vi "Sub_get_freq_bounds_FEA.vi"(2 "FEA Parameters":T1={"LEMP"={"Eigenvalues"=[], "Square Transpose Eigenvectors"=[], "1/deltaStiff"=0.0}, "nodes of interest"=[], "all nodes"=[], "Eigenvalue Method"=enum."0-Local Eigen Modification Procedure", "Mode Count"=3, "initial_pin_node"=0, "Sub Sample"=TRUE}, 3 "Modeling Parameters":T2) -> (0 "FEA Parameters":T1, 1 "Modeling Parameters":T2)   [LabVIEW 2021]
panel:
  out "Waveform Graph":dynamicdata(graph)
  out "third modes":dbl[](array[numeric])
  out "first modes":dbl[](array[numeric])
  out "second modes":dbl[](array[numeric])
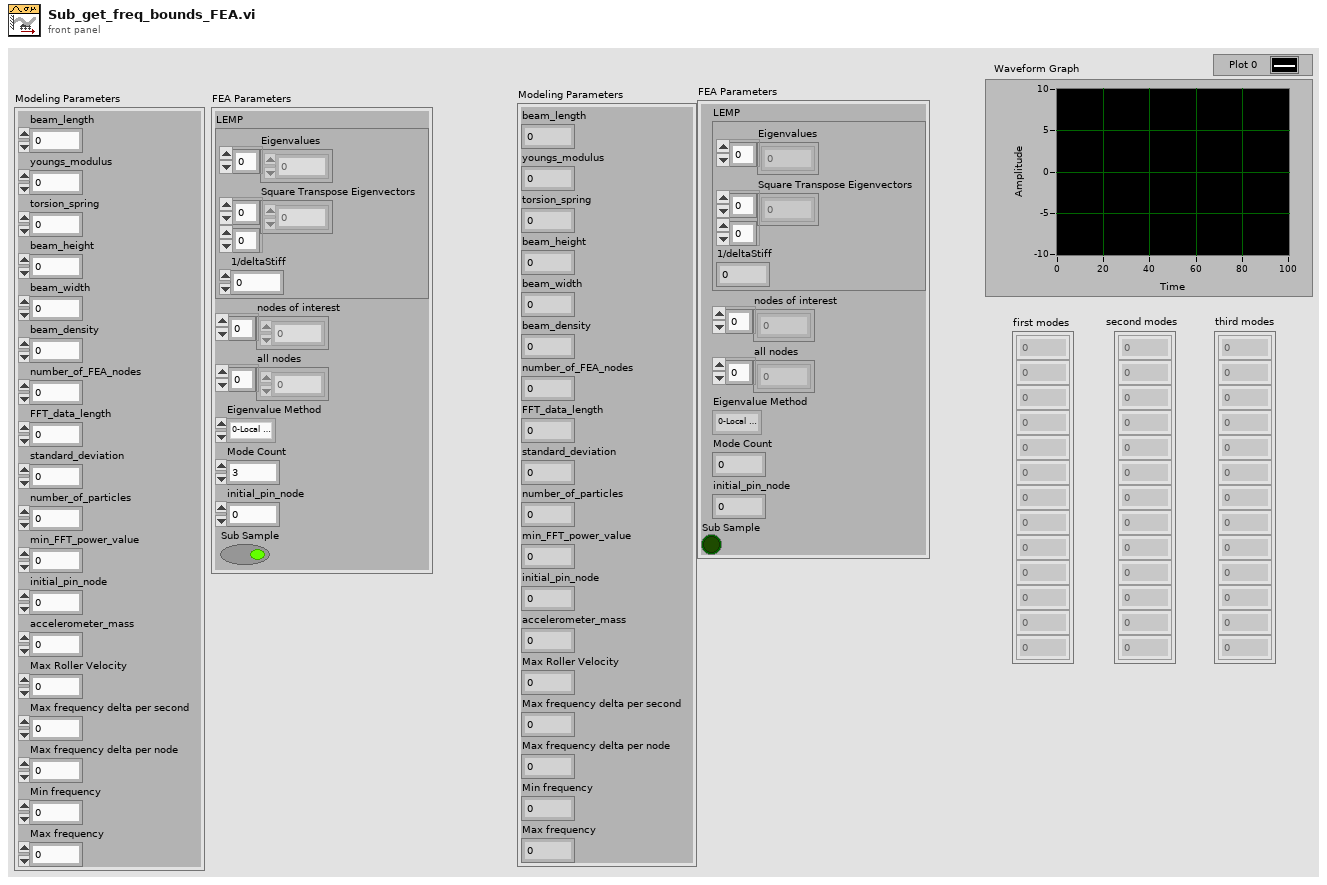
[diagram p1: front panel]
types:
  T1 = cluster{"LEMP":cluster{"Eigenvalues":dbl[], "Square Transpose Eigenvectors":dbl[][], "1/deltaStiff":dbl}, "nodes of interest":i32[], "all nodes":i32[], "Eigenvalue Method":enum16{"0-Local Eigen Modification Procedure", "1-LabVIEW generalized eigenvalues", "2-LabVIEW M^-1K eigenvalues", "3-LabVIEW Cholesky Factorization", "4-Cholesky Factorization CPU SGL", "5-Cholesky Factorization CPU FXP", "6-Cholesky Factorization FPGA SGL", "7-Cholesky Factorization FPGA SGL SCL"}, "Mode Count":i32, "initial_pin_node":i32, "Sub Sample":bool}
  T2 = cluster{"beam_length":dbl, "youngs_modulus":dbl, "torsion_spring":dbl, "beam_height":dbl, "beam_width":dbl, "beam_density":dbl, "number_of_FEA_nodes":i32, "FFT_data_length":i32, "standard_deviation":dbl, "number_of_particles":i32, "min_FFT_power_value":dbl, "initial_pin_node":i32, "accelerometer_mass":dbl, "Max Roller Velocity":dbl, "Max frequency delta per second":dbl, "Max frequency delta per node":dbl, "Min frequency":dbl, "Max frequency":dbl}
  T3 = cluster{"Eigenvalues":dbl[], "Square Transpose Eigenvectors":dbl[][], "1/deltaStiff":dbl}
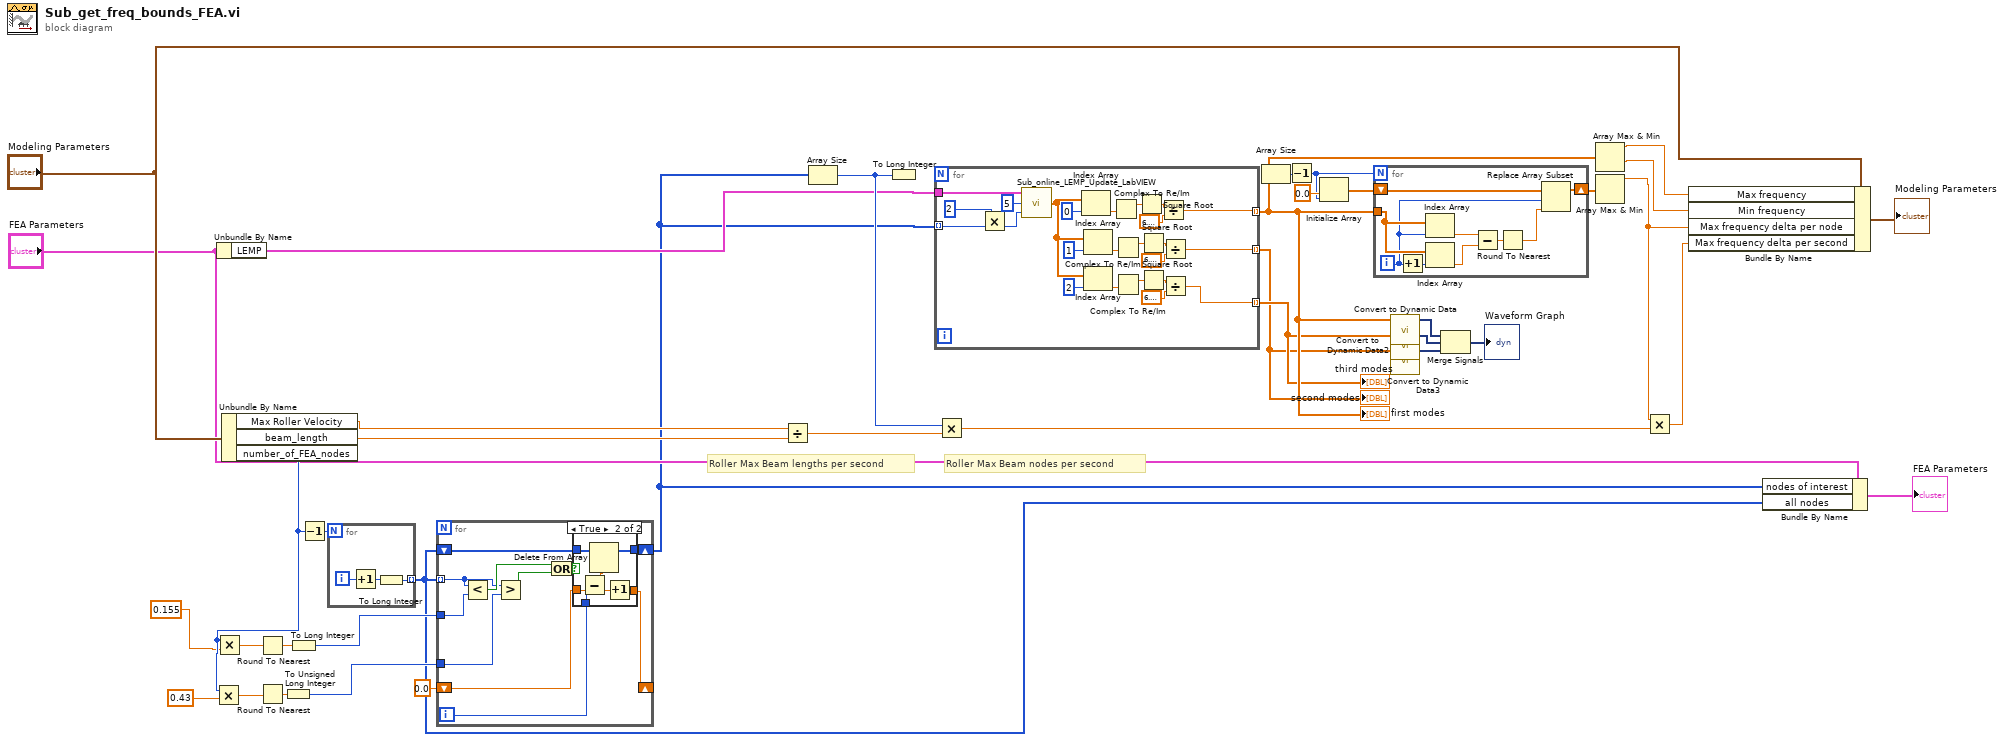
[diagram p0: block diagram]
diagram:
  # "Roller Max Beam nodes per second"
  # "Roller Max Beam lengths per second"
  n1 = Unbundle By Name("FEA Parameters") -> ("LEMP"=w12:T3)
  n2 = Unbundle By Name("Modeling Parameters") -> ("Max Roller Velocity"=w37:dbl, "beam_length"=w36:dbl, "number_of_FEA_nodes"=w29:i32)
  n3 = Multiply(x=w29, y=0.43) -> (x*y=w28:dbl)
  n4 = Multiply(x=w29, y=0.155) -> (x*y=w27:dbl)
  n5 = Round To Nearest(number=w27) -> (nearest integer value=w26:dbl)
  n6 = Round To Nearest(number=w28) -> (nearest integer value=w25:dbl)
  n7 = To Unsigned Long Integer(number=w25) -> (unsigned 32bit integer=w24:u32)
  n8 = To Long Integer(number=w26) -> (32bit integer=w23:i32)
  n9 = Decrement(x=w29) -> (x-1=w33:i32)
  n10 = for {
    N: w33 -> [_]
    tunnel: [w42] -> w19 mode=indexing
    i -> [w40]
    n11 = Increment(x=w40) -> (x+1=w41:i32)
    n12 = To Long Integer(number=w41) -> (32bit integer=w42:i32)
  }
  n13 = for {
    tunnel: w19 -> [w46] mode=indexing
    shift-right: [w49] -> w11
    shift-left: w19 -> [w53]
    shift-right: [w48] -> _
    shift-left: 0.0 -> [w47]
    tunnel: w23 -> [w44]
    tunnel: w24 -> [w43]
    i -> [w45]
    n14 = Less?(x=w46, y=w44) -> (x < y?=w50:bool)
    n15 = Greater?(x=w46, y=w43) -> (0:w52:bool)
    n16 = Or(x=w50, y=w52) -> (x .or. y?=w51:bool)
    n17 = case shown="True" w51 {
      tunnel: w53 -> [w55 w60]
      tunnel: [w55 w61] -> w49
      tunnel: [w54 w59] -> w48
      tunnel: w47 -> [w54 w58]
      tunnel: w45 -> [_ w57]
      frame False {
      }
      frame True {
        n18 = Subtract(x=w57, y=w58) -> (x-y=w56:dbl)
        n19 = Delete From Array(array=w60, index=w56) -> (array with subset deleted=w61:i32[])  [unwired: 1 in, 1 out]
        n20 = Increment(x=w58) -> (x+1=w59:dbl)
      }
    }
  }
  n21 = Divide(x=w37, y=w36) -> (x/y=w39:dbl)
  n22 = Array Size(array=w11) -> (size(s)=w31:i32)
  n23 = To Long Integer(number=w31) -> ()  [unwired: 1 out]
  n24 = for {
    tunnel: w12 -> [w83]
    tunnel: [w76] -> w4 mode=indexing
    tunnel: [w70] -> w2 mode=indexing
    tunnel: [w63] -> w3 mode=indexing
    tunnel: w11 -> [w62] mode=indexing
    n25 = Multiply(x=2, y=w62) -> (x*y=w82:i32)
    n26 = call "Sub_online_LEMP_Update_LabVIEW.vi"("Effected DOF"=w82, "Mode count"=5, "LEMP"=w83) -> ("Updated Eigenvalues"=w64:dbl[])
    n27 = Index Array(array=w64, index=0) -> (element=w80:dbl)
    n28 = Index Array(array=w64, index=1) -> (element=w75:dbl)
    n29 = Index Array(array=w64, index=2) -> (element=w69:dbl)
    n30 = Complex To Re/Im(x + iy=w80) -> (x=w79:dbl)  [unwired: 1 out]
    n31 = Complex To Re/Im(x + iy=w75) -> (x=w74:dbl)  [unwired: 1 out]
    n32 = Complex To Re/Im(x + iy=w69) -> (x=w68:dbl)  [unwired: 1 out]
    n33 = Square Root(x=w79) -> (sqrt(x)=w78:dbl)
    n34 = Square Root(x=w74) -> (sqrt(x)=w73:dbl)
    n35 = Square Root(x=w68) -> (sqrt(x)=w67:dbl)
    n36 = Divide(x=w78, y=6.283185307179586) -> (x/y=w76:dbl)
    n37 = Divide(x=w73, y=6.283185307179586) -> (x/y=w70:dbl)
    n38 = Divide(x=w67, y=6.283185307179586) -> (x/y=w63:dbl)
  }
  "second modes" <- w2
  "first modes" <- w4
  "third modes" <- w3
  n39 = Multiply(x=w31, y=w39) -> (x*y=w38:dbl)
  n40 = Array Size(array=w4) -> (size(s)=w17:i32)
  n41 = Decrement(x=w17) -> (x-1=w14:i32)
  n42 = Initialize Array(0.0 ("element"), w14) -> (w16:dbl[])
  n43 = for {
    N: w14 -> [_]
    tunnel: w4 -> [w94]
    shift-right: [w88] -> w13
    shift-left: w16 -> [w89]
    i -> [w87]
    n44 = Increment(x=w87) -> (x+1=w93:i32)
    n45 = Index Array(array=w94, index=w87) -> (element=w92:dbl)
    n46 = Index Array(array=w94, index=w93) -> (element=w91:dbl)
    n47 = Subtract(x=w92, y=w91) -> (x-y=w90:dbl)
    n48 = Round To Nearest(number=w90) -> (nearest integer value=w86:dbl)
    n49 = Replace Array Subset(array=w89, new element=w86, index=w87) -> (w88:dbl[])
  }
  n50 = call "Convert to Dynamic Data"("Array"=w4) -> ("Dynamic Data Type"=w7:dynamicdata)  [unwired: 3 in]
  n51 = call "Convert to Dynamic Data2"("Array"=w3) -> ("Dynamic Data Type"=w6:dynamicdata)  [unwired: 3 in]
  n52 = call "Convert to Dynamic Data3"("Array"=w2) -> ("Dynamic Data Type"=w5:dynamicdata)  [unwired: 3 in]
  n53 = Merge Signals(w7, w6, w5) -> (→"Waveform Graph":dynamicdata)
  n54 = Array Max & Min(array=w4) -> (max value=w10:dbl, min value=w9:dbl)  [unwired: 2 out]
  n55 = Array Max & Min(array=w13) -> (max value=w8:dbl)  [unwired: 3 out]
  n56 = Multiply(x=w8, y=w38) -> (x*y=w34:dbl)
  n57 = Bundle By Name(cluster="Modeling Parameters", "Max frequency"=w10, "Min frequency"=w9, "Max frequency delta per node"=w8, "Max frequency delta per second"=w34) -> (→"Modeling Parameters":T2)
  n58 = Bundle By Name(cluster="FEA Parameters", "nodes of interest"=w11, "all nodes"=w19) -> (→"FEA Parameters":T1)
